vi "MESADCCheckLotSN.vi"(1 "MES_info":T1={"工号"="2300013", "站别"="F1", "站名"="写信息", "表名称"="test", "工单号"="85255", "条码"="EC82637770B0", "路径"="", "是否连接"="", "电脑名"=""}, 5 "错误输入（无错误）":errorcluster) -> (15 "message":string, 17 "布尔":bool, 19 "错误输出":errorcluster)   [LabVIEW 2014]
uses:
  MES.ctl
  MESControldll.dll
panel:
  out "errbuf":string
  out "POnum":string
  out "m_paramAVal":string
  out "PointGroup 2":string
  out "PointName 2":string
  out "userid 2":string
  out "result 2":i32
  out "POnum 1":i32
  out "result":i32
  # "2300013"
  # "447BBBCDFA60"
  # "MES:CHECK OK"
  # "1001594"
  # "0是代表OK，-1代表NG"
  # "计算机名"
  # "447BBBA1A0D0"
  # "MES:SN [EC82637A4880] \n不允许此测试 [F2]! 当前节点 [F1]"
  # "1001608"
  # "EC8263799B78\nSay{FAIL.wav}请维护规程 [整机维修] 的测试代码!"
  # "85353"
  # "2300013\n447BBBA12C40\n85197\nF6接口测试"
  # "2300013\nEC82637770B0\n85255\nF1信息写入"
  # "2300013\n18132D7F0694\n85174\nF6信息核对"
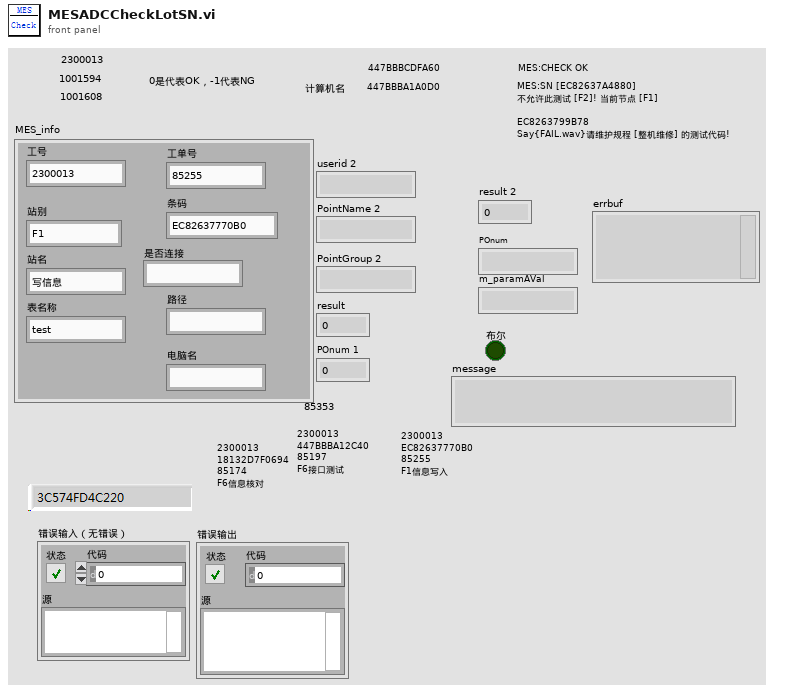
[diagram p1: front panel]
types:
  T1 = typedef "MES.ctl" = cluster{"工号":string, "站别":string, "站名":string, "表名称":string, "工单号":string, "条码":string, "路径":string, "是否连接":string, "电脑名":string}
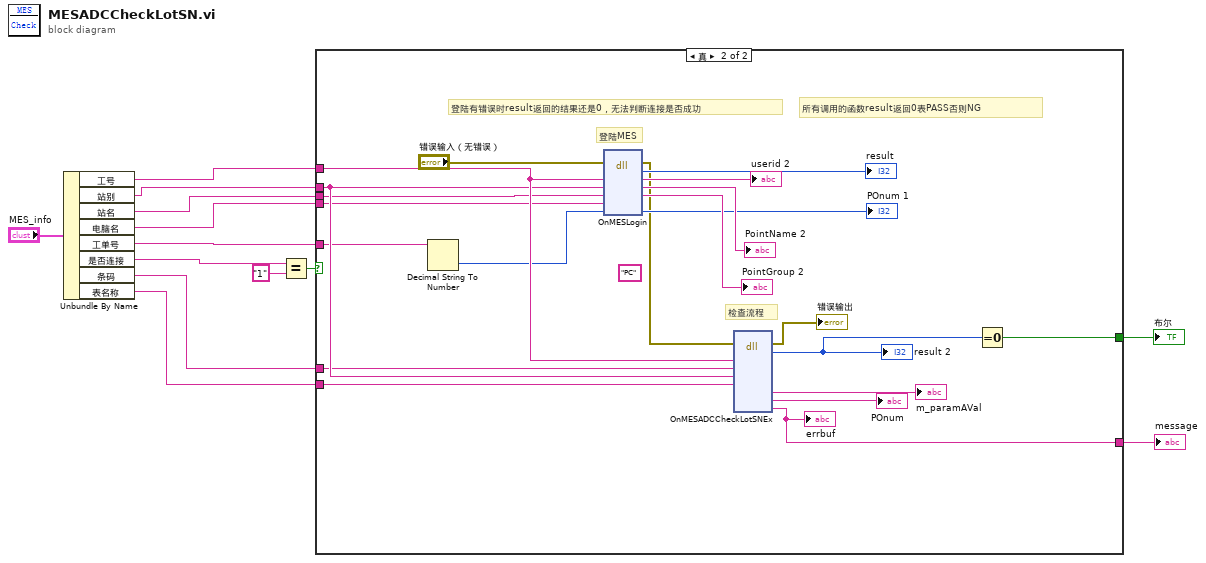
[diagram p0: block diagram]
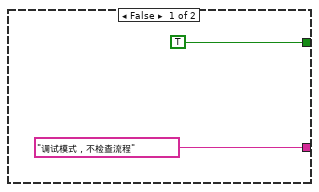
[diagram p2: hidden frame]
diagram:
  n1 = Unbundle By Name("MES_info") -> ("工号"=w2:string, "站别"=w9:string, "站名"=w8:string, "电脑名"=w7:string, "工单号"=w6:string, "是否连接"=w5:string, "条码"=w4:string, "表名称"=w3:string)
  n2 = Equal?(x=w5, y="1") -> (x = y?=w11:bool)
  n3 = case shown="真" w11 {
    tunnel: [TRUE w36] -> w13
    tunnel: ["调试模式，不检查流程" ("key") w35] -> w12
    tunnel: w2 -> [_ w34]
    tunnel: w9 -> [_ w33]
    tunnel: w4 -> [_ w32]
    tunnel: w3 -> [_ w31]
    tunnel: w8 -> [_ w30]
    tunnel: w7 -> [_ w29]
    tunnel: w6 -> [_ w28]
    frame False {
    }
    frame True {
      (unwired) "PC" ("PointPlace")
      # "登陆MES"
      # "检查流程"
      # "登陆有错误时result返回的结果还是0，无法判断连接是否成功"
      # "所有调用的函数result返回0表PASS否则NG"
      n4 = Decimal String To Number(string=w28) -> (number=w18:i32)  [unwired: 2 in, 1 out]
      n5 = dll-call lib="PTH2Dabs CUsers1001563Desktop自写吞吐量MESControldll.dll" fn="OnMESLogin"(error in="错误输入（无错误）", "userid"=w34, "PointName"=w33, "PointGroup"=w30, "PointPlace"=w29, "EquipID"=w18) -> (error out=w17:errorcluster, "result"=→"result":i32, "userid"=→"userid 2":string, "PointName"=→"PointName 2":string, "PointGroup"=→"PointGroup 2":string, "EquipID"=→"POnum 1":i32)  [unwired: 3 in, 1 out]
      n6 = dll-call lib="PTH2Dabs CUsers1001563Desktop自写吞吐量MESControldll.dll" fn="OnMESADCCheckLotSNEx"(error in=w17, "userid"=w34, "barcode"=w32, "pointName"=w33, "pPostCode"=w31) -> (error out=→"错误输出":errorcluster, "result"=w21:i32, "m_paramAVal"=→"m_paramAVal":string, "pszWXPOnum"=→"POnum":string, "errbuf"=w35:string)  [unwired: 9 in, 1 out]
      "result 2" <- w21
      "errbuf" <- w35
      n7 = Equal To 0?(x=w21) -> (x = 0?=w36:bool)
    }
  }
  "布尔" <- w13
  "message" <- w12
